vi "Interpret Signal Strength From Raw Data.vi"   [LabVIEW 2013]
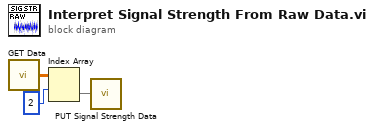
[diagram p0: block diagram]
diagram:
  n1 = call "GET Data.vi"() -> ("Data"=w1:dbl[][])
  n2 = Index Array(array=w1, index (row)=2) -> (element=w2:dbl[])  [unwired: 1 in]
  n3 = call "PUT Signal Strength Data.vi"("Signal Strength Data"=w2) -> ()
